vi "Push.vi"(8 "Error In":errorcluster, 10 "Datum":refnum<class "Abstract.lvclass">, 11 "Context In":refnum<class "Context.lvclass">) -> (0 "Error Out":errorcluster, 3 "Context Out":refnum<class "Context.lvclass">)   [LabVIEW 2018, in "Toolkit.lvlib" / "Data.lvlib" / "Context.lvclass"]
uses:
  Context.lvclass
  Abstract/Abstract.lvclass
  Context.lvclass/Context.ctl
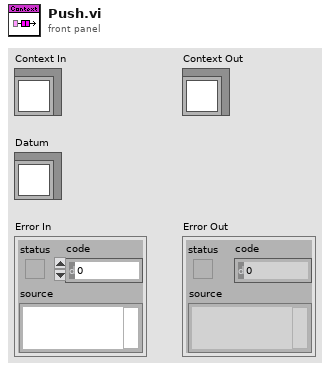
[diagram p1: front panel]
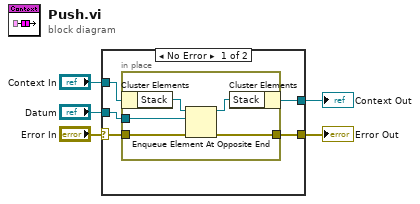
[diagram p0: block diagram]
diagram:
  n1 = case shown="No Error" "Error In" {
    selector: "Error In" -> [w9 w16]
    tunnel: [w7 w16] -> w4
    tunnel: [w8 w17] -> w2
    tunnel: "Context In" -> [w10 w17]
    tunnel: "Datum" -> [w6 _]
    frame No Error {
      n2 = in-place {
        in-place-border: w9 -> [w12]
        in-place-border: [w13] -> w7
        in-place-border: w6 -> [w11]
        n3 = in-place-cluster #1(w10) -> ("Stack"=w15:refnum<queue>)
        n4 = Enqueue Element At Opposite End(queue=w15, element=w11, error in (no error)=w12) -> (queue out=w14:refnum<queue>, error out=w13:errorcluster)  [unwired: 1 in, 1 out]
        n5 = in-place-cluster #1("Stack"=w14) -> (w8:refnum<class "Context.lvclass">)
      }
    }
    frame Error {
    }
  }
  "Error Out" <- w4
  "Context Out" <- w2
